vi "Subvi clipper 4bit.vi"(10 "Input":u8) -> (2 "Output":u8)   [LabVIEW 2017]
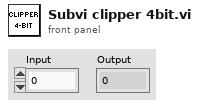
[diagram p1: front panel]
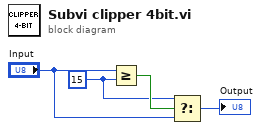
[diagram p0: block diagram]
diagram:
  w2 = u8 15 ("y")
  n1 = Greater Or Equal?(x="Input", y=w2) -> (x >= y?=w4:bool)
  n2 = Select(t=w2, s=w4, f="Input") -> (s? t:f=→"Output":u8)
